vi "NanotecSMCPDDriver.check return string.vi"(2 "expextedReturnString":string, 3 "readString":string) -> (0 "answerValid":bool, 1 "string":string)   [LabVIEW 2014, in "NanotecSMCPDDriver.lvlib"]
doc: "Checks the string that is returned from the serial interface. The string is checked against the expected answer sub-string and the (useful) part of the answer is extracted."
uses:
  NanotecSMCPDDriver.lvlib
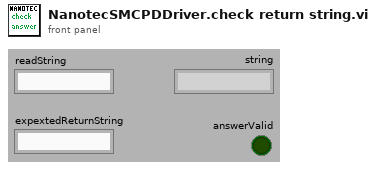
[diagram p1: front panel]
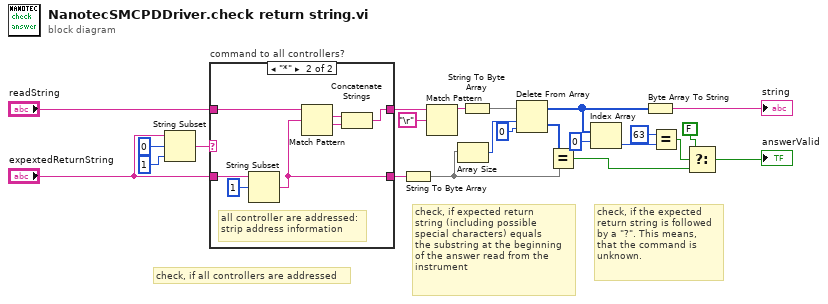
[diagram p0: block diagram]
diagram:
  # "check, if all controllers are addressed"
  # "check, if the expected\nreturn string is followed\nby a \"?\". This means,\nthat the command is\nunknown."
  # "check, if expected return\nstring (including possible \nspecial characters) equals\nthe substring at the beginning\nof the answer read from the\ninstrument"
  n1 = String Subset(string="expextedReturnString", offset (0)=0, length (rest)=1 ("length (rest)")) -> (substring=w5:string)
  n2 = case "command to all controllers?" shown="\"*\"" w5 {
    tunnel: [w25 w29] -> w3
    tunnel: "expextedReturnString" -> [w25 w31]
    tunnel: [w24 w28] -> w1
    tunnel: "readString" -> [w24 w30]
    frame Default {
    }
    frame "*" {
      # "all controller are addressed:\nstrip address information"
      n3 = String Subset(string=w31, offset (0)=1) -> (substring=w29:string)  [unwired: 1 in]
      n4 = Match Pattern(string=w30, regular expression=w29) -> (match substring=w27:string, after substring=w26:string)  [unwired: 1 in, 2 out]
      n5 = Concatenate Strings(w27, w26) -> (w28:string)
    }
  }
  n6 = String To Byte Array(string=w3) -> (unsigned byte array=w9:u8[])
  n7 = Match Pattern(string=w1, regular expression="\r") -> (before substring=w15:string)  [unwired: 1 in, 3 out]
  n8 = Array Size(array=w9) -> (size(s)=w17:i32)
  n9 = String To Byte Array(string=w15) -> (unsigned byte array=w16:u8[])
  n10 = Delete From Array(array=w16, length=w17, index=0) -> (deleted portion=w19:u8[], array with subset deleted=w13:u8[])
  n11 = Equal?(x=w19, y=w9) -> (x = y?=w7:bool)
  n12 = Index Array(array=w13, index=0) -> (element=w11:u8)
  n13 = Byte Array To String(unsigned byte array=w13) -> (string=→"string":string)
  n14 = Equal?(x=u8 63, y=w11) -> (x = y?=w8:bool)
  n15 = Select(t=FALSE, s=w8, f=w7) -> (s? t:f=→"answerValid":bool)
